vi "DI Bank A Injection.vi"(8 "error in":errorcluster, 9 "Device Inputs":dbl[](array[numeric]), 10 "DCM Ref":refnum<class "DCM - RT.lvclass">, 11 "DI-A Cmd in":T1={"DI Command Enabled"=FALSE, "Sync Pump Enabled"=FALSE, "FIFO Indexes"={"Write"={"DI Command"=[], "Pump Command"={"Mode"=-1, "Digital Input"=-1, "Default Profile Index"=-1, "Cal Freq [Hz]"=-1, "Cal Duration [s]"=-1, "Cal Increment [s]"=-1, "Cal Pulses"=-1, "TMP Command Sequence"=[{"Duration [s]"=-1, "Level"=-1, "Run/Stop"=-1, "Profile Index"=-1}, {"Duration [s]"=-1, "Level"=-1, "Run/Stop"=-1, "Profile Index"=-1}, {"Duration [s]"=-1, "Level"=-1, "Run/Stop"=-1, "Profile Index"=-1}, {"Duration [s]"=-1, "Level"=-1, "Run/Stop"=-1, "Profile Index"=-1}, {"Duration [s]"=-1, "Level"=-1, "Run/Stop"=-1, "Profile Index"=-1}, {"Duration [s]"=-1, "Level"=-1, "Run/Stop"=-1, "Profile Index"=-1}, {"Duration [s]"=-1, "Level"=-1, "Run/Stop"=-1, "Profile Index"=-1}, {"Duration [s]"=-1, "Level"=-1, "Run/Stop"=-1, "Profile Index"=-1}], "EPT TDC Offset [CAD]"=-1, "EPT Window Start [DBTDC]"=-1, "EPT Window End [DBTDC]"=-1, "EPT Angles"=[{"Enable"=-1, "Timing [DBTDC]"=-1, "Duration [s]"=-1, "Profile Index"=-1}, {"Enable"=-1, "Timing [DBTDC]"=-1, "Duration [s]"=-1, "Profile Index"=-1}, {"Enable"=-1, "Timing [DBTDC]"=-1, "Duration [s]"=-1, "Profile Index"=-1}, {"Enable"=-1, "Timing [DBTDC]"=-1, "Duration [s]"=-1, "Profile Index"=-1}], "EPT Skip Fire"=-1, "EPT Skip Index"=-1, "EPT Precharge Duration [s]"=-1, "EPT Precharge Profile Index"=-1}}}, "Settings"={"Inj Phase Arrays"=[], "Pump Phase Array"=[], "Pulsewidths [s]"=[]}} {"Settings"."Pump Phase Array"."Profile" max=15; "Settings"."Pump Phase Array"."Period [s]" min=0 max=0.000102 format="%#_3p"; "Settings"."Pump Phase Array"."Pulse Width [s]" min=0 max=0.000102 format="%#_3p"; "Settings"."Pump Phase Array"."Voltage Low [V]" min=-250 max=250 format="%#_3p"; "Settings"."Pump Phase Array"."Voltage High [V]" min=-250 max=250 format="%#_3p"; "Settings"."Pump Phase Array"."Current Low [A]" min=-40 max=40 format="%#_3p"; "Settings"."Pump Phase Array"."Current High [A]" min=-40 max=40 format="%#_3p"; "Settings"."Pump Phase Array"."Duration [s]" min=0 max=1.67772 format="%#_3p"; "Settings"."Inj Phase Arrays"."Profile" max=15; "Settings"."Inj Phase Arrays"."Period [s]" min=0 max=0.000102 format="%#_3p"; "Settings"."Inj Phase Arrays"."Pulse Width [s]" min=0 max=0.000102 format="%#_3p"; "Settings"."Inj Phase Arrays"."Voltage Low [V]" min=-250 max=250 format="%#_3p"; "Settings"."Inj Phase Arrays"."Voltage High [V]" min=-250 max=250 format="%#_3p"; "Settings"."Inj Phase Arrays"."Current Low [A]" min=-40 max=40 format="%#_3p"; "Settings"."Inj Phase Arrays"."Current High [A]" min=-40 max=40 format="%#_3p"; "Settings"."Inj Phase Arrays"."Duration [s]" min=0 max=1.67772 format="%#_3p"}) -> (0 "error out":errorcluster)   [LabVIEW 2016, in "DCM Engine.lvlib"]
uses:
  DCM Engine.lvlib
  Built/DCM Classes Packed/Pharlap/C/DCM-Classes.lvlibp/DCM/Rev0/RT/DCM - RT.lvclass
  Shared/Types/DI.ctl
  Shared/Types/DI Command Indexes.ctl
  Shared/Types/DI Phase Outputs.ctl
  <vilib>/Powertrain Controls/Device Drivers/DCM/DI/RT/Phase.ctl
  <vilib>/Powertrain Controls/Device Drivers/DCM/Rev0/FPGA/DI - Drive State.ctl
  <vilib>/Powertrain Controls/Device Drivers/DCM/DI/FPGA/Phase Step.ctl
  <vilib>/Powertrain Controls/Device Drivers/DCM/DI/FPGA/Control.ctl
  Built/DCM Classes Packed/Pharlap/C/DCM-Classes.lvlibp/DCM/DI/RT/DCM - RT - DI.lvlib
  DCM Shared.lvlib
  <vilib>/Powertrain Controls/Device Drivers/DCM/DI/RT/DCM - RT - DI.lvlib
  <vilib>/Powertrain Controls/Device Drivers/DCM/Rev0/FPGA/DCM - FPGA.lvlib
  <vilib>/Powertrain Controls/Device Drivers/DCM/DI/FPGA/DCM - FPGA - DI.lvlib
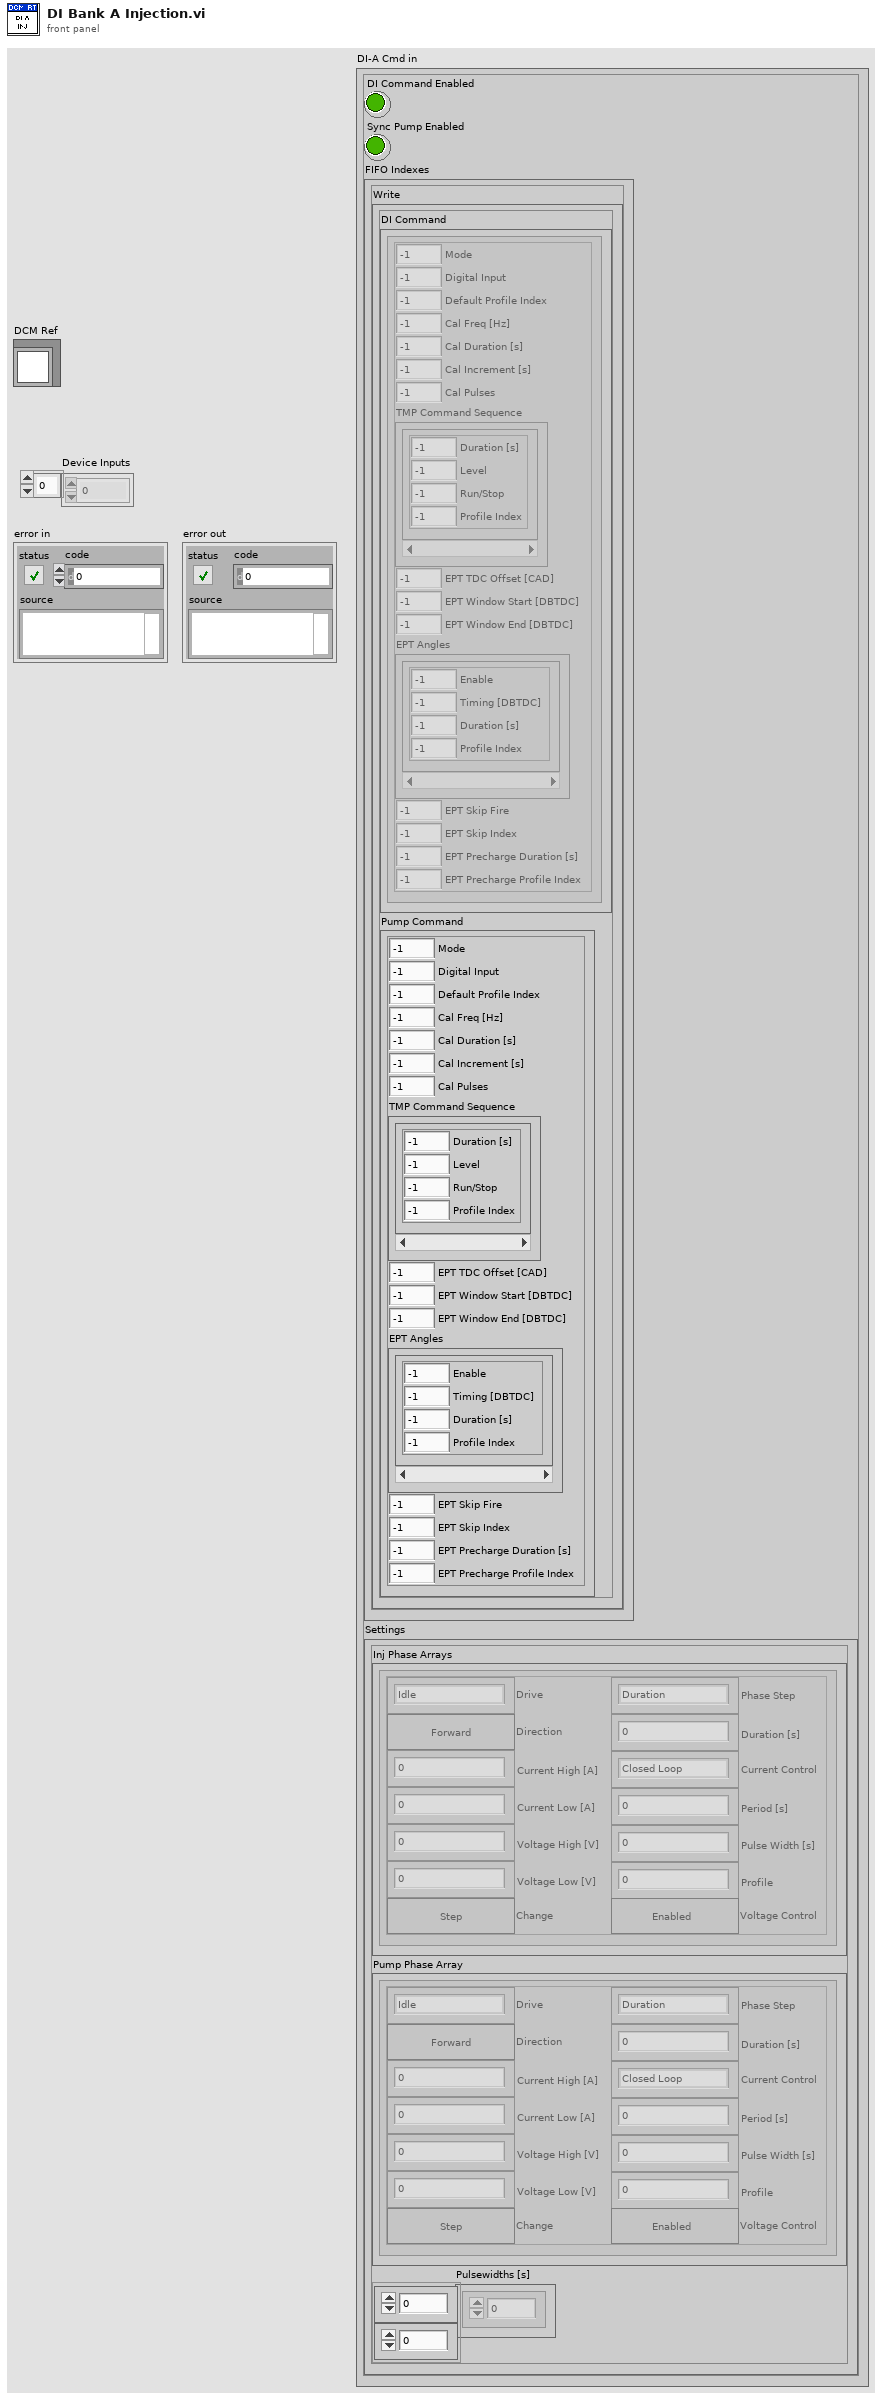
[diagram p1: front panel]
types:
  T1 = typedef "DCM Shared.lvlib/DI.ctl" = cluster{"DI Command Enabled":bool, "Sync Pump Enabled":bool, "FIFO Indexes":cluster{"Write":cluster{"DI Command":T2[], "Pump Command":T2}}, "Settings":T3}
  T2 = typedef "DCM Shared.lvlib/DI Command Indexes.ctl" = cluster{"Mode":i32, "Digital Input":i32, "Default Profile Index":i32, "Cal Freq [Hz]":i32, "Cal Duration [s]":i32, "Cal Increment [s]":i32, "Cal Pulses":i32, "TMP Command Sequence":cluster{"Duration [s]":i32, "Level":i32, "Run/Stop":i32, "Profile Index":i32}[], "EPT TDC Offset [CAD]":i32, "EPT Window Start [DBTDC]":i32, "EPT Window End [DBTDC]":i32, "EPT Angles":cluster{"Enable":i32, "Timing [DBTDC]":i32, "Duration [s]":i32, "Profile Index":i32}[], "EPT Skip Fire":i32, "EPT Skip Index":i32, "EPT Precharge Duration [s]":i32, "EPT Precharge Profile Index":i32}
  T3 = typedef "DCM Shared.lvlib/DI Phase Outputs.ctl" = cluster{"Inj Phase Arrays":T4[][], "Pump Phase Array":T4[], "Pulsewidths [s]":sgl[][]}
  T4 = typedef "DCM - RT - DI.lvlib/Phase.ctl" = cluster{"Drive":T5, "Direction":bool, "Phase Step":T6, "Duration [s]":sgl, "Current High [A]":sgl, "Current Low [A]":sgl, "Voltage High [V]":sgl, "Voltage Low [V]":sgl, "Change":bool, "Current Control":T7, "Period [s]":sgl, "Pulse Width [s]":sgl, "Profile":u8, "Voltage Control":bool}
  T5 = typedef "DCM - FPGA.lvlib/DI - Drive State.ctl" = enum8{"Idle", "HV Current Control", "LV Current Control", "Back Boost", "Piezo Charge", "Piezo Discharge"}
  T6 = typedef "DCM - FPGA - DI.lvlib/Phase Step.ctl" = enum8{"Duration", "First Peak", "End of Cmd", "Branch", "2-Phase Duration"}
  T7 = typedef "DCM - FPGA - DI.lvlib/Control.ctl" = enum8{"Closed Loop", "Fixed Period", "Fixed On Pulse", "Fixed Off Pulse", "Open Loop", "Profile"}
  T8 = typedef "DCM-Classes.lvlibp/DCM - RT - DI.lvlib/Command.ctl" = cluster{"Mode":T9, "Digital Input":T10, "Default Profile Index":u8, "Cal Freq [Hz]":sgl, "Cal Duration [s]":sgl, "Cal Increment [s]":sgl, "Cal Pulses":u16, "TMP Command Sequence":T11[], "EPT TDC Offset [CAD]":sgl, "EPT Window Start [DBTDC]":sgl, "EPT Window End [DBTDC]":sgl, "EPT Angles":T12[], "EPT Skip Fire":bool, "EPT Skip Index":u8, "EPT Precharge Duration [s]":sgl, "EPT Precharge Profile Index":u8}
  T9 = typedef "DCM-Classes.lvlibp/DCM - FPGA - DI.lvlib/Mode.ctl" = enum8{"Off", "Direct", "Calibration", "Triggered Multi-Pulse", "Engine Position Tracking"}
  T10 = typedef "DCM-Classes.lvlibp/DCM - FPGA.lvlib/Digital Channel.ctl" = enum8{"Unused", "User OS", "Diff IO 1", "Diff IO 2", "Diff IO 3", "Diff IO 4", "Diff IO 5", "Diff IO 6", "Diff IO 7", "Diff IO 8", "Aux 1", "Aux 2", "Aux 3", "Aux 4", "Aux 5", "Aux 6", "Aux 7", "Aux 8", "Aux 9", "Aux 10", "Aux 11", "Aux 12", "Aux 13", "Aux 14", "Aux 15", "Aux 16"}
  T11 = typedef "DCM-Classes.lvlibp/DCM - RT - DI.lvlib/Command Sequence.ctl" = cluster{"Duration [s]":sgl, "Level":bool, "Run/Stop":bool, "Profile Index":u8}
  T12 = typedef "DCM-Classes.lvlibp/DCM - RT - DI.lvlib/Angle Control.ctl" = cluster{"Enable":bool, "Timing [DBTDC]":sgl, "Duration [s]":sgl, "Profile Index":u8}
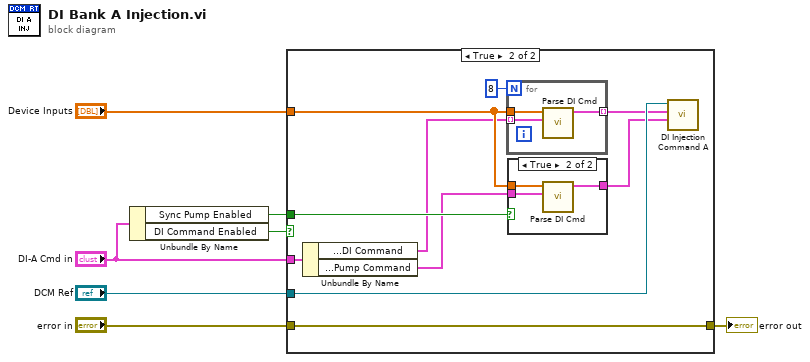
[diagram p0: block diagram]
diagram:
  n1 = Unbundle By Name("DI-A Cmd in") -> ("Sync Pump Enabled"=w2:bool, "DI Command Enabled"=w1:bool)
  n2 = case shown="True" w1 {
    tunnel: "error in" -> [w8 w18]
    tunnel: "DCM Ref" -> [_ w14]
    tunnel: [w8 w18] -> w5
    tunnel: "Device Inputs" -> [_ w17]
    tunnel: "DI-A Cmd in" -> [_ w16]
    tunnel: w2 -> [_ w15]
    frame False {
    }
    frame True {
      n3 = Unbundle By Name(w16) -> ("FIFO Indexes.Write.DI Command"=w13:T2[], "FIFO Indexes.Write.Pump Command"=w12:T2)
      n4 = for {
        N: 8 -> [_]
        tunnel: w13 -> [w23] mode=indexing
        tunnel: [w24] -> w9 mode=indexing
        tunnel: w17 -> [w22]
        n5 = call "Parse DI Cmd.vi"("FIFO Indexes"=w23, "Device Inputs"=w22) -> ("Injection Setup out"=w24:T8)  [unwired: 9 in]
      }
      n6 = case shown="True" w15 {
        tunnel: w17 -> [_ w21]
        tunnel: w12 -> [_ w20]
        tunnel: [_ w19] -> w11
        frame False {
        }
        frame True {
          n7 = call "Parse DI Cmd.vi"("FIFO Indexes"=w20, "Device Inputs"=w21) -> ("Injection Setup out"=w19:T8)  [unwired: 9 in]
        }
      }
      n8 = call "DI Injection Command A.vi"("A Pump Command"=w11, "A DI Command"=w9, "DCM Reference"=w14) -> ()  [unwired: 9 in]
    }
  }
  "error out" <- w5
